vi "Begin.vi"(8 "error in":errorcluster) -> (0 "error out":errorcluster)   [LabVIEW 2020]
doc: "Called before other user functions, this VI is expected to open initial I/O refnums, load in file data, and do all program initialization. Notice that the <B>error out</B> terminal is simply used for data flow. Wiring it to other structures or subVIs ensures that this VI runs first."
uses:
  <vilib>/Rock Robotics/WPI/DriverStation/WPI_DriverStationRobotMode2.ctl
  <vilib>/Rock Robotics/WPI/Joystick/WPI_JoystickDeviceEnum.ctl
  <vilib>/Rock Robotics/WPI/ThirdParty/REV Robotics/REVLib/Typedef/Spark MAX Control Type.ctl
  <vilib>/Rock Robotics/WPI/ThirdParty/Sensors/navX/_TypeDefs/FRIC_navX_DeviceNumbersTypeDef.ctl
  Robot Global Data.vi
  <vilib>/Rock Robotics/Network Tables/NT Write String Array.vi
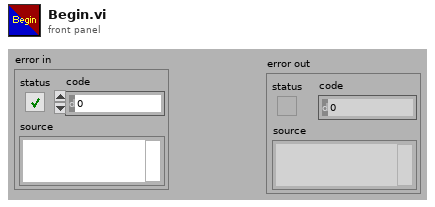
[diagram p1: front panel]
types:
  T1 = typedef "FRIC_navX_DeviceNumbersTypeDef.ctl" = enum16{"Dev0", "Dev1", "Dev2", "Dev3"}
  T2 = typedef "Spark MAX Control Type.ctl" = enum16{"Percent VBus", "Voltage", "Velocity", "Position", "Smart Motion", "Current", "Smart Velocity"}
  T3 = typedef "WPI_JoystickDeviceEnum.ctl" = enum16{"USB 0", "USB 1", "USB 2", "USB 3", "USB 4", "USB 5"}
  T4 = typedef "WPI_DriverStationRobotMode2.ctl" = enum16{"Autonomous Disabled", "Autonomous Enabled", "Teleop Disabled", "Teleop Enabled", "Disconnected", "Finish", "Test Disabled", "Test Enabled", "Emergency Stopped"}
  T5 = typedef "WPI_JoystickDevRef.ctl" = cluster{"Device":T3}
  T6 = typedef "WPI_MotorControlDeviceRef.ctl" = cluster{"DeviceStatus":errorcluster, "Type":T7, "PWM":cluster{"PWM Channel":T8, "DeadBand":T9}, "CAN":cluster{"Device Number":u8, "SetOutput VI Ref":variant, "GetOutput VI Ref":variant, "Enable VI Ref":variant, "Disable VI Ref":variant, "Data":variant}, "Invert":bool, "DIO PWM":cluster{"PWM \"Enable\" Channel":T8, "DIOChannel":T10, "PWM Rate":dbl}}
  T7 = typedef "WPI_MotorControlType.ctl" = enum16{"PWM", "CAN", "DIO PWM"}
  T8 = typedef "FPGA_DIOPWMChannel.ctl" = enum8{"PWM 0", "PWM 1", "PWM 2", "PWM 3", "PWM 4", "PWM 5", "PWM 6", "PWM 7", "PWM 8", "PWM 9", "PWM MXP 0", "PWM MXP 1", "PWM MXP 2", "PWM MXP 3", "PWM MXP 4", "PWM MXP 5", "PWM MXP 6", "PWM MXP 7", "PWM MXP 8", "PWM MXP 9", "Invalid"}
  T9 = typedef "WPI_PWMDeadband.ctl" = cluster{"Name":string, "maxPositivePwm":i32, "minPositivePwm":i32, "centerPwm":i32, "maxNegativePwm":i32, "minNegativePwm":i32, "angularRange":u16}
  T10 = typedef "FPGA_DIOChannel.ctl" = enum8{"DIO 0", "DIO 1", "DIO 2", "DIO 3", "DIO 4", "DIO 5", "DIO 6", "DIO 7", "DIO 8", "DIO 9", "DIO MXP 0", "DIO MXP 1", "DIO MXP 2", "DIO MXP 3", "DIO MXP 4", "DIO MXP 5", "DIO MXP 6", "DIO MXP 7", "DIO MXP 8", "DIO MXP 9", "DIO MXP 10", "DIO MXP 11", "DIO MXP 12", "DIO MXP 13", "DIO MXP 14", "DIO MXP 15", "SPI Port CS1", "SPI Port CS2", "SPI Port CS3", "SPI Port MISO", "SPI Port MOSI", "Invalid"}
  T11 = typedef "CTRE_Phoenix_CANcoder_DeviceRef.ctl" = cluster{"DeviceStatus":errorcluster, "Device Number":u8, "Handle":u64, "UsageFrame":u32, "Library Path":path}
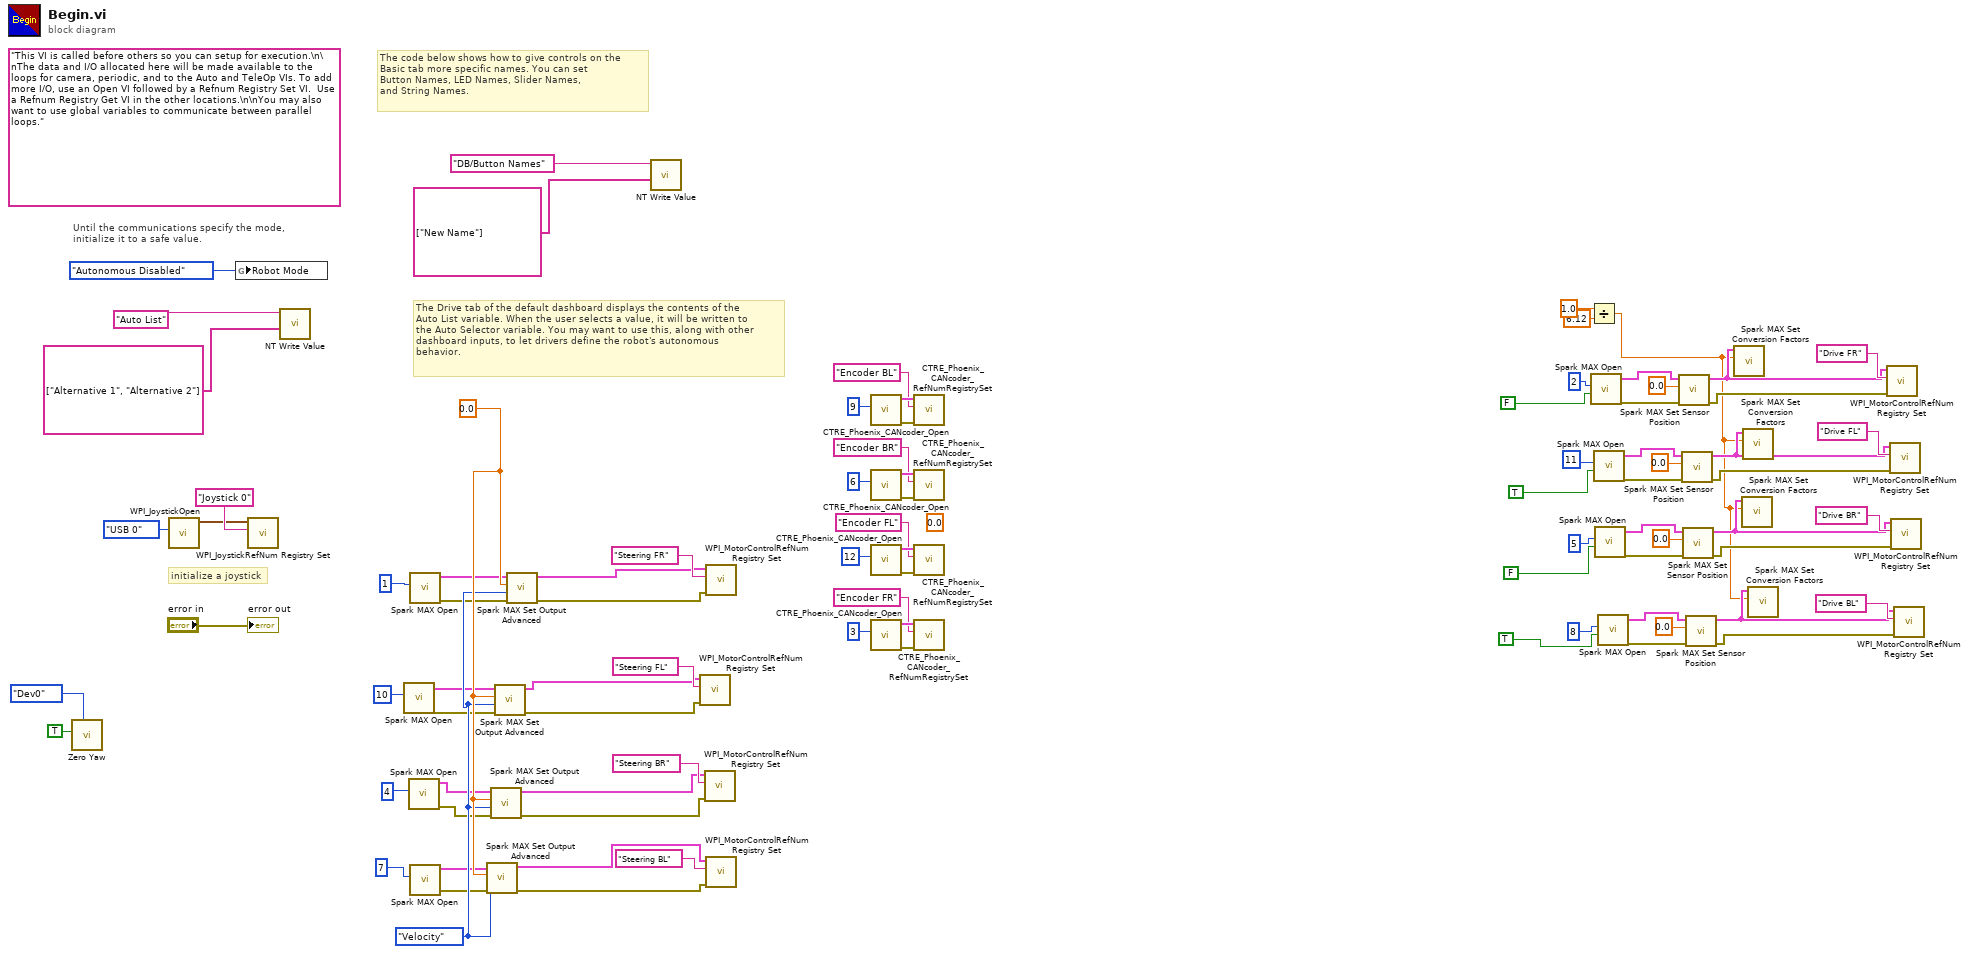
[diagram p0: block diagram]
diagram:
  w30 = Spark_MAX_Control_Type."Velocity" ("Control Mode")
  (unwired) 0.0 ("Position")
  w31 = 0.0 ("New Position")
  (unwired) "This VI is called before others so you can setup for execution.\n\nThe data and I/O allocated here will be made available to the loops for camera, periodic, and to the Auto and TeleOp VIs. To add more I/O, use an Open VI followed by a Refnum Registry Set VI.  Use a Refnum Registry Get VI in the other locations.\n\nYou may also want to use global variables to communicate between parallel loops."
  # "The Drive tab of the default dashboard displays the contents of the\nAuto List variable. When the user selects a value, it will be written to\nthe Auto Selector variable. You may want to use this, along with other\ndashboard inputs, to let drivers define the robot's autonomous\nbehavior."
  # "The code below shows how to give controls on the\nBasic tab more specific names. You can set\nButton Names, LED Names, Slider Names,\nand String Names."
  # "initialize a joystick"
  # "Until the communications specify the mode,\ninitialize it to a safe value."
  n1 = call <vilib>:"Zero Yaw.vi"("Device Number"=FRIC_navX_DeviceNumbersTypeDef."Dev0", "Zero"=TRUE) -> ()  [unwired: 10 in]
  n2 = call <vilib>:"WPI_JoystickOpen.vi"("JoystickDevice"=WPI_JoystickDeviceEnum."USB 0") -> ("JoystickDevRef"=w86:T5)  [unwired: 10 in]
  n3 = global write "Robot Global Data.vi" "Robot Mode"(WPI_DriverStationRobotMode2."Autonomous Disabled" ("Robot Mode")) -> ()
  n4 = call <vilib>:"WPI_JoystickRefNum Registry Set.vi"("refnum name"="Joystick 0", "JoystickDevRef"=w86) -> ()  [unwired: 8 in, 2 out]
  n5 = call-poly <vilib>:"NT Write Value.vi"("value"=string[] ["Alternative 1", "Alternative 2"] ("String Array"), "name"="Auto List" ("Name")) -> ()  [unwired: 9 in, 1 out]
  n6 = call <vilib>:"Spark MAX Open.vi"("Device Number"=u8 10) -> ("error out"=w26:errorcluster, "MotorControlDeviceRef"=w27:T6)  [unwired: 9 in]
  n7 = call <vilib>:"Spark MAX Open.vi"("Device Number"=u8 4) -> ("error out"=w24:errorcluster, "MotorControlDeviceRef"=w25:T6)  [unwired: 9 in]
  n8 = call <vilib>:"Spark MAX Open.vi"("Device Number"=u8 1) -> ("error out"=w28:errorcluster, "MotorControlDeviceRef"=w29:T6)  [unwired: 9 in]
  n9 = call <vilib>:"Spark MAX Open.vi"("Device Number"=u8 7) -> ("error out"=w22:errorcluster, "MotorControlDeviceRef"=w23:T6)  [unwired: 9 in]
  n10 = call <vilib>:"Spark MAX Set Output Advanced.vi"("error in (no error)"=w22, "Control Mode"=w30, "Setpoint"=w31, "MotorControlDevRef"=w23) -> ("error out"=w20:errorcluster, "MotorControlDevRef"=w21:T6)  [unwired: 6 in]
  n11 = call <vilib>:"Spark MAX Set Output Advanced.vi"("error in (no error)"=w24, "Control Mode"=w30, "Setpoint"=w31, "MotorControlDevRef"=w25) -> ("error out"=w18:errorcluster, "MotorControlDevRef"=w19:T6)  [unwired: 6 in]
  n12 = call <vilib>:"Spark MAX Set Output Advanced.vi"("error in (no error)"=w26, "Control Mode"=w30, "Setpoint"=w31, "MotorControlDevRef"=w27) -> ("error out"=w16:errorcluster, "MotorControlDevRef"=w17:T6)  [unwired: 6 in]
  n13 = call <vilib>:"Spark MAX Set Output Advanced.vi"("error in (no error)"=w28, "Control Mode"=w30, "Setpoint"=w31, "MotorControlDevRef"=w29) -> ("error out"=w14:errorcluster, "MotorControlDevRef"=w15:T6)  [unwired: 6 in]
  n14 = call-poly <vilib>:"NT Write Value.vi"("value"=string[] ["New Name"], "name"="DB/Button Names" ("Name")) -> ()  [unwired: 9 in, 1 out]
  n15 = call <vilib>:"WPI_MotorControlRefNum Registry Set.vi"("error in (no error)"=w16, "refnum name"="Steering FL", "MotorControlDevRef"=w17) -> ()  [unwired: 7 in, 2 out]
  n16 = call <vilib>:"WPI_MotorControlRefNum Registry Set.vi"("error in (no error)"=w18, "refnum name"="Steering BR", "MotorControlDevRef"=w19) -> ()  [unwired: 7 in, 2 out]
  n17 = call <vilib>:"WPI_MotorControlRefNum Registry Set.vi"("error in (no error)"=w14, "refnum name"="Steering FR", "MotorControlDevRef"=w15) -> ()  [unwired: 7 in, 2 out]
  n18 = call <vilib>:"WPI_MotorControlRefNum Registry Set.vi"("error in (no error)"=w20, "refnum name"="Steering BL", "MotorControlDevRef"=w21) -> ()  [unwired: 7 in, 2 out]
  n19 = call <vilib>:"CTRE_Phoenix_CANcoder_Open.vi"("Device Number"=u8 9) -> ("error out"=w67:errorcluster, "CTRE_CANcoder_DeviceRef"=w66:T11)  [unwired: 9 in]
  n20 = call <vilib>:"CTRE_Phoenix_CANcoder_Open.vi"("Device Number"=u8 6) -> ("error out"=w71:errorcluster, "CTRE_CANcoder_DeviceRef"=w70:T11)  [unwired: 9 in]
  n21 = call <vilib>:"CTRE_Phoenix_CANcoder_Open.vi"("Device Number"=u8 12) -> ("error out"=w75:errorcluster, "CTRE_CANcoder_DeviceRef"=w74:T11)  [unwired: 9 in]
  n22 = call <vilib>:"CTRE_Phoenix_CANcoder_Open.vi"("Device Number"=u8 3) -> ("error out"=w79:errorcluster, "CTRE_CANcoder_DeviceRef"=w78:T11)  [unwired: 9 in]
  n23 = call <vilib>:"CTRE_Phoenix_CANcoder_RefNumRegistrySet.vi"("error in (no error)"=w67, "refnum name"="Encoder BL", "CTRE_CANcoder_DeviceRef"=w66) -> ()  [unwired: 7 in, 2 out]
  n24 = call <vilib>:"CTRE_Phoenix_CANcoder_RefNumRegistrySet.vi"("error in (no error)"=w71, "refnum name"="Encoder BR", "CTRE_CANcoder_DeviceRef"=w70) -> ()  [unwired: 7 in, 2 out]
  n25 = call <vilib>:"CTRE_Phoenix_CANcoder_RefNumRegistrySet.vi"("error in (no error)"=w75, "refnum name"="Encoder FL", "CTRE_CANcoder_DeviceRef"=w74) -> ()  [unwired: 7 in, 2 out]
  n26 = call <vilib>:"CTRE_Phoenix_CANcoder_RefNumRegistrySet.vi"("error in (no error)"=w79, "refnum name"="Encoder FR", "CTRE_CANcoder_DeviceRef"=w78) -> ()  [unwired: 7 in, 2 out]
  n27 = Divide(x=1.0, y=6.12) -> (x/y=w1:dbl)
  n28 = call <vilib>:"Spark MAX Open.vi"("Invert"=FALSE, "Device Number"=u8 2) -> ("error out"=w53:errorcluster, "MotorControlDeviceRef"=w54:T6)  [unwired: 8 in]
  n29 = call <vilib>:"Spark MAX Open.vi"("Invert"=TRUE, "Device Number"=u8 11) -> ("error out"=w49:errorcluster, "MotorControlDeviceRef"=w50:T6)  [unwired: 8 in]
  n30 = call <vilib>:"Spark MAX Open.vi"("Invert"=FALSE, "Device Number"=u8 5) -> ("error out"=w45:errorcluster, "MotorControlDeviceRef"=w46:T6)  [unwired: 8 in]
  n31 = call <vilib>:"Spark MAX Open.vi"("Invert"=TRUE, "Device Number"=u8 8) -> ("error out"=w41:errorcluster, "MotorControlDeviceRef"=w42:T6)  [unwired: 8 in]
  n32 = call <vilib>:"Spark MAX Set Sensor Position.vi"("error in"=w53, "Position"=0.0 ("New Position"), "MotorControlDeviceRef"=w54) -> ("error out"=w52:errorcluster, "MotorControlDeviceRef"=w4:T6)  [unwired: 7 in]
  n33 = call <vilib>:"Spark MAX Set Sensor Position.vi"("error in"=w49, "Position"=0.0 ("New Position"), "MotorControlDeviceRef"=w50) -> ("error out"=w48:errorcluster, "MotorControlDeviceRef"=w5:T6)  [unwired: 7 in]
  n34 = call <vilib>:"Spark MAX Set Sensor Position.vi"("error in"=w45, "Position"=0.0 ("New Position"), "MotorControlDeviceRef"=w46) -> ("error out"=w44:errorcluster, "MotorControlDeviceRef"=w6:T6)  [unwired: 7 in]
  n35 = call <vilib>:"Spark MAX Set Sensor Position.vi"("error in"=w41, "Position"=0.0 ("New Position"), "MotorControlDeviceRef"=w42) -> ("error out"=w40:errorcluster, "MotorControlDeviceRef"=w7:T6)  [unwired: 7 in]
  n36 = call <vilib>:"Spark MAX Set Conversion Factors.vi"("Position Factor (1)"=w1, "MotorControlDeviceRef in"=w4) -> ()  [unwired: 8 in, 2 out]
  n37 = call <vilib>:"Spark MAX Set Conversion Factors.vi"("Position Factor (1)"=w1, "MotorControlDeviceRef in"=w6) -> ()  [unwired: 8 in, 2 out]
  n38 = call <vilib>:"Spark MAX Set Conversion Factors.vi"("Position Factor (1)"=w1, "MotorControlDeviceRef in"=w5) -> ()  [unwired: 8 in, 2 out]
  n39 = call <vilib>:"Spark MAX Set Conversion Factors.vi"("Position Factor (1)"=w1, "MotorControlDeviceRef in"=w7) -> ()  [unwired: 8 in, 2 out]
  n40 = call <vilib>:"WPI_MotorControlRefNum Registry Set.vi"("error in (no error)"=w52, "refnum name"="Drive FR", "MotorControlDevRef"=w4) -> ()  [unwired: 7 in, 2 out]
  n41 = call <vilib>:"WPI_MotorControlRefNum Registry Set.vi"("error in (no error)"=w48, "refnum name"="Drive FL", "MotorControlDevRef"=w5) -> ()  [unwired: 7 in, 2 out]
  n42 = call <vilib>:"WPI_MotorControlRefNum Registry Set.vi"("error in (no error)"=w44, "refnum name"="Drive BR", "MotorControlDevRef"=w6) -> ()  [unwired: 7 in, 2 out]
  n43 = call <vilib>:"WPI_MotorControlRefNum Registry Set.vi"("error in (no error)"=w40, "refnum name"="Drive BL", "MotorControlDevRef"=w7) -> ()  [unwired: 7 in, 2 out]
  "error out" <- "error in"
